vi "Besoin_fond_de_roulement.vi"(1 "Argent ventes":dbl, 2 "dettes":dbl) -> (0 "BFR":dbl)   [LabVIEW 2024]
uses:
  Stock_MP.vi
  Prix_MP.vi
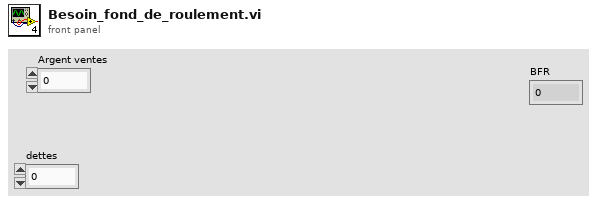
[diagram p1: front panel]
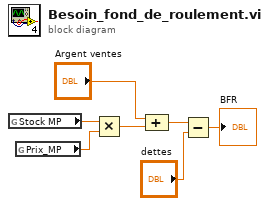
[diagram p0: block diagram]
diagram:
  n1 = global read "Stock_MP.vi" "Stock MP"() -> (w3:dbl)
  n2 = global read "Prix_MP.vi" "Prix_MP"() -> (w2:dbl)
  n3 = Multiply(x=w3, y=w2) -> (x*y=w1:dbl)
  n4 = Compound Arithmetic op=ADD("Argent ventes", w1) -> (w5:dbl)
  n5 = Subtract(x=w5, y="dettes") -> (x-y=→"BFR":dbl)
